vi "Read Timebase.vi"(8 "error in (no error)":errorcluster, 11 "NiPxi6733 in":refnum<class "NiPxi6733.lvclass">) -> (0 "error out":errorcluster, 2 "Timebase":cluster{"Src":tag, "Rate":dbl}={"Src"="/PXI1Slot6/PXI_Star", "Rate"=20000000.0} {"Rate" format="%#_6p"}, 3 "NiPxi6733 out":refnum<class "NiPxi6733.lvclass">)   [LabVIEW 2014, in "FGenPlugins.lvlib" / "NiPxi6733.lvclass"]
uses:
  NiPxi6733.lvclass
  NiPxi6733.lvclass/NiPxi6733.ctl
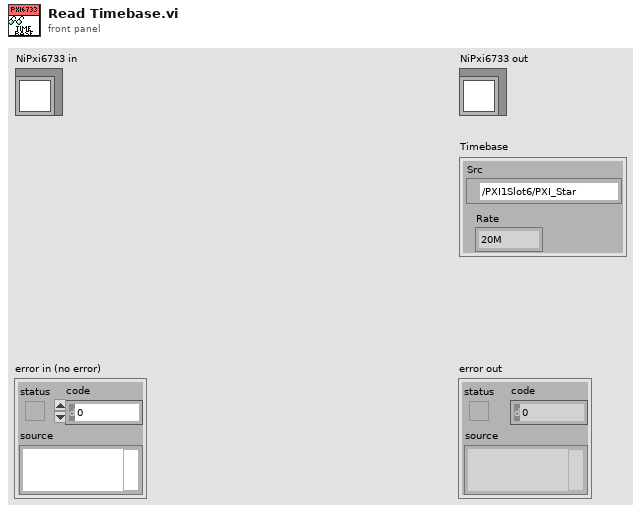
[diagram p1: front panel]
types:
  T1 = typedef "FGenPlugins.lvlib/NiPxi6733.lvclass/clTimebase.ctl" = cluster{"Src":tag, "Rate":dbl}
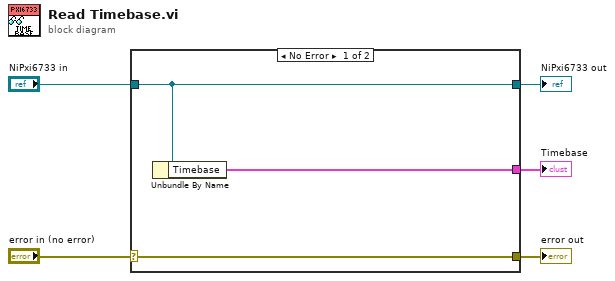
[diagram p0: block diagram]
diagram:
  n1 = case shown="No Error" "error in (no error)" {
    selector: "error in (no error)" -> [w8 w9]
    tunnel: [w8 w9] -> w4
    tunnel: [w7 w10] -> w2
    tunnel: "NiPxi6733 in" -> [w7 w10]
    tunnel: [w6 _] -> w1
    frame No Error {
      n2 = Unbundle By Name(w7) -> ("Timebase"=w6:T1)
    }
    frame Error {
    }
  }
  "error out" <- w4
  "NiPxi6733 out" <- w2
  "Timebase" <- w1
